vi "PCO_TIMESTAMP_STRUCT.vi"() -> (0 "PCO_TIMESTAMP_STRUCT":T1 {"lvTimestamp" format="%<%.6X\n%x>T"}, 1 "PCO_TIMESTAMP_STRUCT_Raw":T2, 2 "Length":u16, 3 "Raw_Length":u16)   [LabVIEW 2020, in "SDK.lvlib" / "Structures.lvlib"]
doc: "Use this template to build a VI to use as a subVI."
uses:
  Structures.lvlib
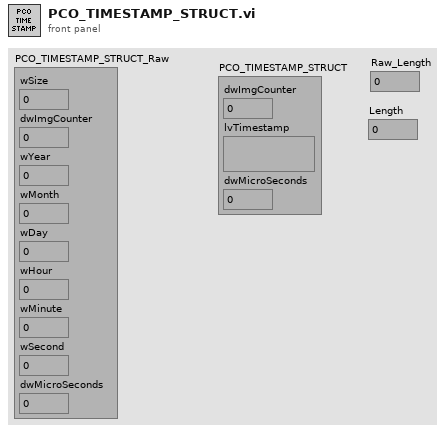
[diagram p1: front panel]
types:
  T1 = cluster{"dwImgCounter":u32, "lvTimestamp":timestamp, "dwMicroSeconds":u32}
  T2 = cluster{"wSize":u16, "dwImgCounter":u32, "wYear":u16, "wMonth":u16, "wDay":u16, "wHour":u16, "wMinute":u16, "wSecond":u16, "dwMicroSeconds":u32}
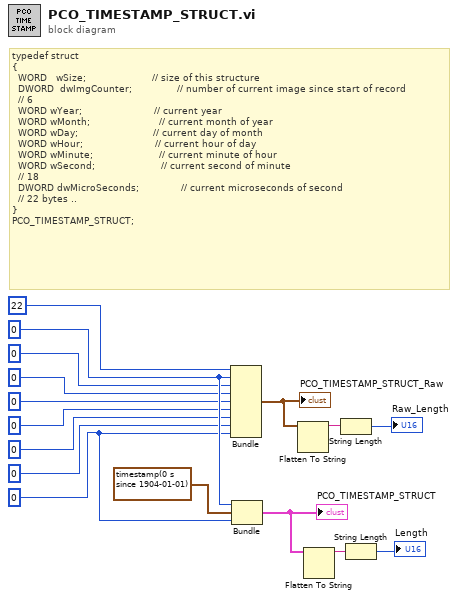
[diagram p0: block diagram]
diagram:
  w2 = u32 0 ("dwMicroSeconds")
  w9 = u32 0 ("dwImgCounter")
  # "typedef struct\n{\n  WORD   wSize;                      // size of this structure\n  DWORD  dwImgCounter;               // number of current image since start of record\n  // 6\n  WORD wYear;                        // current year\n  WORD wMonth;                       // current month of year\n  WORD wDay;                         // current day of month\n  WORD wHour;                        // current hour of day\n  WORD wMinute;                      // current minute of hour\n  WORD wSecond;                      // current second of minute\n  // 18\n  DWORD dwMicroSeconds;              // current microseconds of second\n  // 22 bytes ..\n}\nPCO_TIMESTAMP_STRUCT;"
  n1 = Bundle("wSize"=u16 22, "dwImgCounter"=w9, "wYear"=u16 0, "wMonth"=u16 0, "wDay"=u16 0, "wHour"=u16 0, "wMinute"=u16 0, "wSecond"=u16 0, "dwMicroSeconds"=w2) -> (w11:T2)  [unwired: 1 in]
  "PCO_TIMESTAMP_STRUCT_Raw" <- w11
  n2 = Bundle("dwImgCounter"=w9, "lvTimestamp"=timestamp(0 s since 1904-01-01), "dwMicroSeconds"=w2) -> (w10:T1)  [unwired: 1 in]
  "PCO_TIMESTAMP_STRUCT" <- w10
  n3 = Flatten To String(anything=w11) -> (data string=w15:string)  [unwired: 3 in, 2 out]
  n4 = Flatten To String(anything=w10) -> (data string=w16:string)  [unwired: 3 in, 2 out]
  n5 = String Length(string=w15) -> (length=→"Raw_Length":i32)
  n6 = String Length(string=w16) -> (length=→"Length":i32)
